vi "Circuito1.vi"() -> ()   [LabVIEW 2019]
panel:
  out "dB":dbl
  in  "Potencia 2":dbl
  in  "Potencia 1":dbl
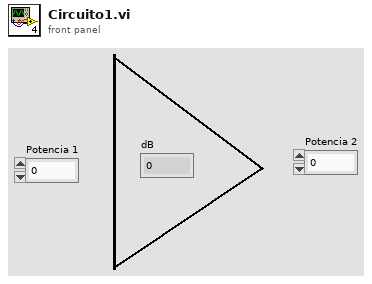
[diagram p1: front panel]
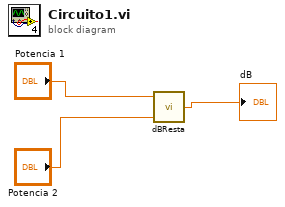
[diagram p0: block diagram]
diagram:
  n1 = call "dBResta.vi"("Potencia Salida"="Potencia 2", "Potencia Entrada"="Potencia 1") -> ("dB"=→"dB":dbl)  [unwired: 2 in, 1 out]
